vi "Inventory-PullInventoryTree.vi"(7 "Raw Data From DB Actor":string[][](array[string])=[["1", "tej", "2/28/13", "3/15/2013", "123456987987", "This is a dummy test", "50", "dummy instructions", "unassigned", "2/28/13", "1234556"], ["2", "tej", "2/28/13", "1/25/2013", "123456987987", "This is a dummy test", "50", "dummy instructions", "unassigned", "2/28/13", "1234556"], ["4", "tej", "2/28/13", "3/25/2013", "123456987987", "This is a dummy test", "50", "dummy instructions", "unassigned", "2/28/13", "1234556"], ["6", "tej", "2/28/13", "12/05/2012", "123456987987", "This is a dummy test", "50", "dummy instructions", "unassigned", "2/28/13", "1234556"]], 8 "error in (no error)":errorcluster, 11 "ERP-Inventory in":refnum<class "ERP-Inventory.lvclass">) -> (0 "error out":errorcluster, 3 "ERP-Inventory out":refnum<class "ERP-Inventory.lvclass">)   [LabVIEW 2013, in "ERP-Inventory.lvclass"]
uses:
  ERP-Inventory.lvclass
  ERP-Inventory.lvclass/ERP-Inventory.ctl
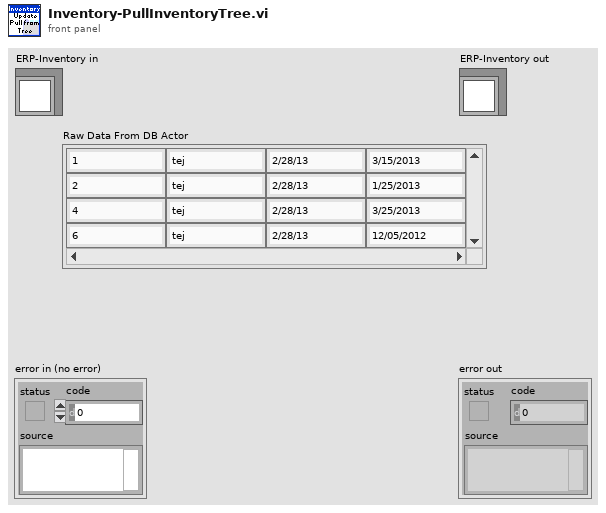
[diagram p1: front panel]
types:
  T1 = typedef "imagedata.ctl" = cluster{"image type":i32, "image depth":i32, "image":u8[], "mask":u8[], "colors":u32[], "Rectangle":cluster{"left":i16, "top":i16, "right":i16, "bottom":i16}}
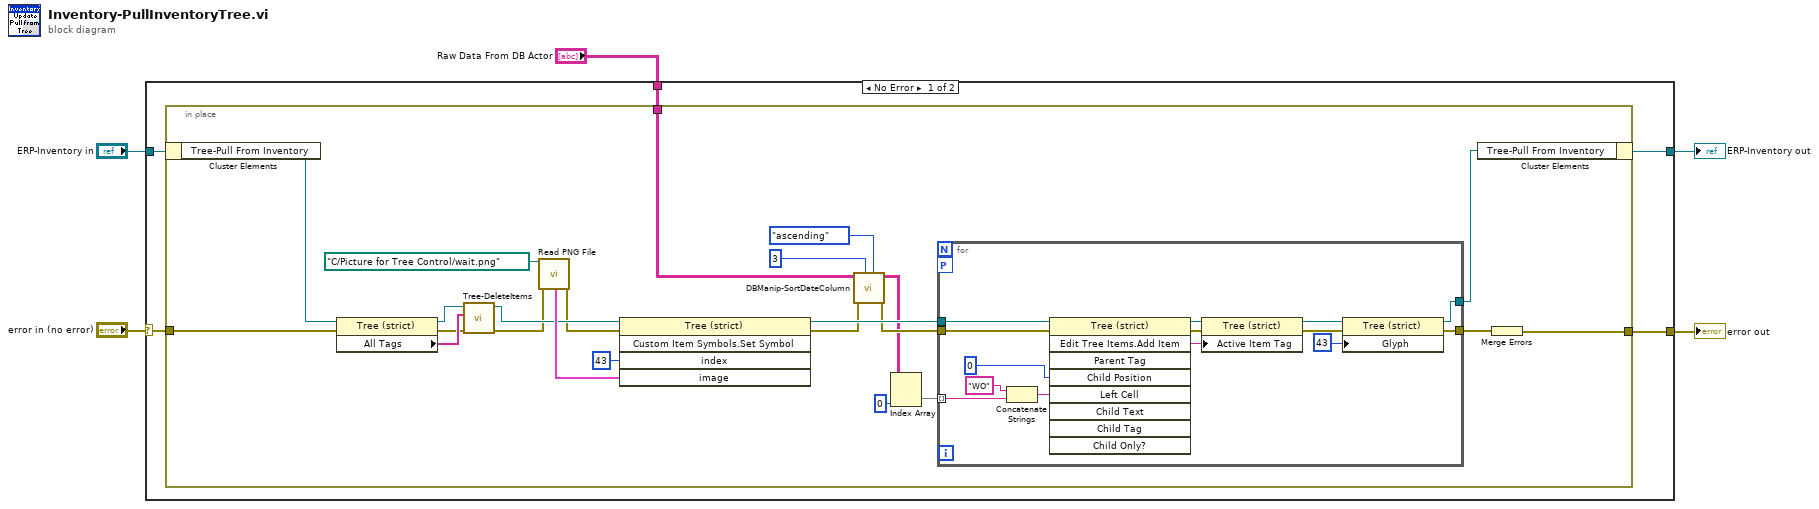
[diagram p0: block diagram]
diagram:
  n1 = case shown="No Error" "error in (no error)" {
    selector: "error in (no error)" -> [w10 w48]
    tunnel: [w7 w49] -> w3
    tunnel: "ERP-Inventory in" -> [w8 w49]
    tunnel: [w9 w48] -> w2
    tunnel: "Raw Data From DB Actor" -> [w6 _]
    frame No Error {
      n2 = in-place {
        in-place-border: w10 -> [w25]
        in-place-border: [w15] -> w9
        in-place-border: w6 -> [w11]
        n3 = in-place-cluster #1(w8) -> ("Tree-Pull From Inventory"=w14:refnum<vi>)
        n4 = property class="Tree (strict)"(reference=w14, error in=w25) -> (reference out=w23:refnum<vi>, error out=w21:errorcluster, "All Tags"=w24:string[])
        n5 = call "Tree-DeleteItems.vi"("error In"=w21, "All Tags"=w24, "Tree In"=w23) -> ("error out"=w20:errorcluster, "Tree out"=w22:refnum<vi>)  [unwired: 7 in]
        n6 = call <vilib>:"Read PNG File.vi"("error in (no error)"=w20, "path to PNG file"=path "C:/Picture for Tree Control/wait.png") -> ("error out"=w19:errorcluster, "image data"=w32:T1)  [unwired: 7 in, 1 out]
        n7 = invoke class="Tree (strict)" method="Custom Item Symbols.Set Symbol"(reference=w22, error in=w19, "index"=43 ("Index"), "image"=w32) -> (reference out=w33:refnum<vi>, error out=w28:errorcluster)  [unwired: 1 in, 3 out]
        n8 = call "DBManip-SortDateColumn.vi"("Sorting Order"=enum16{"ascending", "descending"}."ascending", "disabled index (col)"=3, "error in"=w28, "DB Table Data"=w11) -> ("error out"=w27:errorcluster, "Sorted Data by Date"=w18:string[][])  [unwired: 6 in]
        n9 = Index Array(array=w18, index (col)=0 ("disabled index (col)")) -> (element=w29:string[])  [unwired: 1 in]
        n10 = for {
          tunnel: w33 -> [w44]
          tunnel: w27 -> [w45]
          tunnel: [w47] -> w13
          tunnel: [w46] -> w16
          tunnel: w29 -> [w34] mode=indexing
          workers-P: _ -> [_]
          n11 = Concatenate Strings("WO" ("string"), w34) -> (w42:string)
          n12 = invoke class="Tree (strict)" method="Edit Tree Items.Add Item"(reference=w44, error in=w45, "Child Position"=0, "Left Cell"=w42) -> (reference out=w38:refnum<vi>, error out=w39:errorcluster, "Edit Tree Items:Add Item"=w41:string)  [unwired: 5 in, 6 out]
          n13 = property class="Tree (strict)"(reference=w38, error in=w39, "Active Item Tag"=w41) -> (reference out=w36:refnum<vi>, error out=w37:errorcluster)
          n14 = property class="Tree (strict)"(reference=w36, error in=w37, "Glyph"=43 ("Active Item:Symbol Index")) -> (reference out=w47:refnum<vi>, error out=w46:errorcluster)
        }
        n15 = in-place-cluster #1("Tree-Pull From Inventory"=w13) -> (w7:refnum<class "ERP-Inventory.lvclass">)
        n16 = Merge Errors(w16) -> (w15:errorcluster)
      }
    }
    frame Error {
    }
  }
  "error out" <- w2
  "ERP-Inventory out" <- w3
